vi "dfd_Convert FXP info to MRate Filter.vi"(8 "error in (no error)":errorcluster, 10 "xml string in":string, 11 "multirate filter in":T1={"mMRate_Structure"=enum."CIC", "mMRate_Mode"=0, "mMRate_Factor"=1, "mMRate_FIRParams"={"mMRate_FIR_H"=[], "mMRate_FIR_IsNyquist?"=FALSE, "mMRate_FIR_IsSymmetric?"=FALSE}, "mMRate_CICParams"={"mMRate_CIC_#Stage"=2, "mMRate_CIC_Lag"=1, "mMRate_CIC_Type"=enum."Lowpass"}, "mMRate_Order"=1, "mMRate_Version"="1.0", "mMRate_Comments"="1.0", "mMRate_RationalFactor"={"mMRate_L"=-1, "mMRate_M"=-1}, "mMRate_Fs"=0.0, "mMRate_Quantized?"=FALSE, "mMRate_QFilterGain"=1.0, "mMRate_CoefWl"=16, "mMRate_Scaling"={"mMRate_ScaleByPowerOf2?"=FALSE, "mMRate_ScaleType"=enum."Time Domain 1-Norm"}, "mMRate_InputWl"=0, "mMRate_OutputWl"=0, "mMRate_OutputMode"=enum."Nearest", "mMRate_MultMode"=enum."Truncated", "mMRate_BitPruning"=FALSE, "mMRate_GainWl"=16, "mMRate_OutputFwl"=0, "mMRate_SumIwl"=0, "mMRate_InputIwl "=16, "mMRate_SumWl"=32, "mMRate_CoefIwl"=0} {"mMRate_SumWl" min=1 max=32 step=1; "mMRate_InputIwl" min=1 max=32 step=1; "mMRate_GainWl" min=1 max=32 step=1; "mMRate_OutputWl" min=1 max=32 step=1; "mMRate_InputWl" min=1 max=32 step=1; "mMRate_CoefWl" min=1 max=32 step=1; "mMRate_Mode" items=["Default"=-1, "No Rate Change"=0, "Interpolation"=1, "Decimation"=2, "Interpolated"=3, "Rational"=4]}) -> (0 "error out":errorcluster, 3 "multirate filter out":T1={"mMRate_Structure"=enum."IIR", "mMRate_Mode"=0, "mMRate_Factor"=-1, "mMRate_FIRParams"={"mMRate_FIR_H"=[], "mMRate_FIR_IsNyquist?"=FALSE, "mMRate_FIR_IsSymmetric?"=FALSE}, "mMRate_CICParams"={"mMRate_CIC_#Stage"=0, "mMRate_CIC_Lag"=0, "mMRate_CIC_Type"=enum."Lowpass"}, "mMRate_Order"=0, "mMRate_Version"="2.0", "mMRate_Comments"="", "mMRate_RationalFactor"={"mMRate_L"=-1, "mMRate_M"=-1}, "mMRate_Fs"=1.0, "mMRate_Quantized?"=FALSE, "mMRate_QFilterGain"=1.0, "mMRate_CoefWl"=16, "mMRate_Scaling"={"mMRate_ScaleByPowerOf2?"=FALSE, "mMRate_ScaleType"=enum."No Norm"}, "mMRate_InputWl"=16, "mMRate_OutputWl"=16, "mMRate_OutputMode"=enum."Truncation", "mMRate_MultMode"=enum."Truncated", "mMRate_BitPruning"=FALSE, "mMRate_GainWl"=16, "mMRate_OutputFwl"=0, "mMRate_SumIwl"=0, "mMRate_InputIwl "=16, "mMRate_SumWl"=32, "mMRate_CoefIwl"=0} {"mMRate_SumWl" min=1 max=32 step=1; "mMRate_InputIwl" min=1 max=32 step=1; "mMRate_GainWl" min=1 max=32 step=1; "mMRate_OutputWl" min=1 max=32 step=1; "mMRate_InputWl" min=1 max=32 step=1; "mMRate_CoefWl" min=1 max=32 step=1; "mMRate_Mode" items=["Default"=-1, "No Rate Change"=0, "Interpolation"=1, "Decimation"=2, "Interpolated"=3, "Rational"=4]})   [LabVIEW 2017, in "NI_DigFilter_Process.lvlib"]
uses:
  <vilib>/addons/Digital Filter Design/NI_DigFilter_Process.lvlib
  <vilib>/addons/Digital Filter Design/_Objects.llb/DFD Multirate Filter Obj.ctl
  <vilib>/addons/Digital Filter Design/_Objects.llb/DFD Multirate Mode.ctl
  <vilib>/addons/Digital Filter Design/_Objects.llb/DFD Coef Norm Type.ctl
  <vilib>/addons/Digital Filter Design/_Objects.llb/DFD Round-off Mode.ctl
  <vilib>/addons/Digital Filter Design/_Objects.llb/DFD FXP MRate Multiply Mode.ctl
  <vilib>/addons/Digital Filter Design/_Objects.llb/DFD Quantization Settings.ctl
  <vilib>/addons/Digital Filter Design/_Objects.llb/DFD Quantization Sources.ctl
  <vilib>/addons/Digital Filter Design/FXPLib.llb/DFD I32 to FXP (scalar).vi
  <vilib>/addons/Digital Filter Design/NI_DigFilterLicensed.lvlib
panel:
  in  "Q settings":T6={"source"=0, "wl"=16, "iwl"=1, "overflow mode"=enum."Wrap", "rounding mode"=enum."Truncation", "signed?"=TRUE} {"source" items=["Coefficients a/k"=0, "Coefficients b/v"=7, "Input"=1, "Output"=2, "Multiplicand"=3, "Product"=4, "Sum"=5, "Delay"=6]}
  in  "Q settings":T6={"source"=0, "wl"=16, "iwl"=1, "overflow mode"=enum."Wrap", "rounding mode"=enum."Truncation", "signed?"=TRUE} {"source" items=["Coefficients a/k"=0, "Coefficients b/v"=7, "Input"=1, "Output"=2, "Multiplicand"=3, "Product"=4, "Sum"=5, "Delay"=6]}
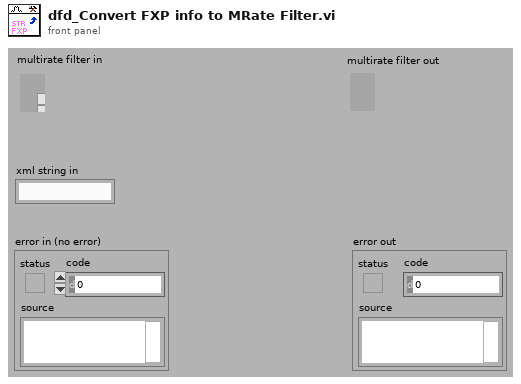
[diagram p1: front panel]
types:
  T1 = typedef "NI_DigFilterLicensed.lvlib/DFD Multirate Filter Obj.ctl" = cluster{"mMRate_Structure":enum16{"CIC", "FIR", "IIR", "Lattice"}, "mMRate_Mode":T2, "mMRate_Factor":i32, "mMRate_FIRParams":cluster{"mMRate_FIR_H":dbl[], "mMRate_FIR_IsNyquist?":bool, "mMRate_FIR_IsSymmetric?":bool}, "mMRate_CICParams":cluster{"mMRate_CIC_#Stage":i32, "mMRate_CIC_Lag":i32, "mMRate_CIC_Type":enum16{"Lowpass", "Highpass"}}, "mMRate_Order":i32, "mMRate_Version":string, "mMRate_Comments":string, "mMRate_RationalFactor":cluster{"mMRate_L":i32, "mMRate_M":i32}, "mMRate_Fs":dbl, "mMRate_Quantized?":bool, "mMRate_QFilterGain":dbl, "mMRate_CoefWl":i16, "mMRate_Scaling":cluster{"mMRate_ScaleByPowerOf2?":bool, "mMRate_ScaleType":T3}, "mMRate_InputWl":i16, "mMRate_OutputWl":i16, "mMRate_OutputMode":T4, "mMRate_MultMode":T5, "mMRate_BitPruning":bool, "mMRate_GainWl":i16, "mMRate_OutputFwl":i16, "mMRate_SumIwl":i16, "mMRate_InputIwl ":i16, "mMRate_SumWl":i16, "mMRate_CoefIwl":i16}
  T2 = typedef "NI_DigFilterLicensed.lvlib/DFD Multirate Mode.ctl" = i16
  T3 = typedef "NI_DigFilterLicensed.lvlib/DFD Coef Norm Type.ctl" = enum16{"No Norm", "Time Domain 1-Norm", "Time Domain 2-Norm", "Time Domain Inf-Norm"}
  T4 = typedef "NI_DigFilterLicensed.lvlib/DFD Round-off Mode.ctl" = enum16{"Nearest", "Truncation"}
  T5 = typedef "NI_DigFilterLicensed.lvlib/DFD FXP MRate Multiply Mode.ctl" = enum16{"Truncated", "Full"}
  T6 = typedef "NI_DigFilterLicensed.lvlib/DFD Quantization Settings.ctl" = cluster{"source":T7, "wl":i16, "iwl":i16, "overflow mode":enum16{"Saturation", "Wrap"}, "rounding mode":enum16{"Nearest", "Truncation"}, "signed?":bool}
  T7 = typedef "NI_DigFilterLicensed.lvlib/DFD Quantization Sources.ctl" = u16
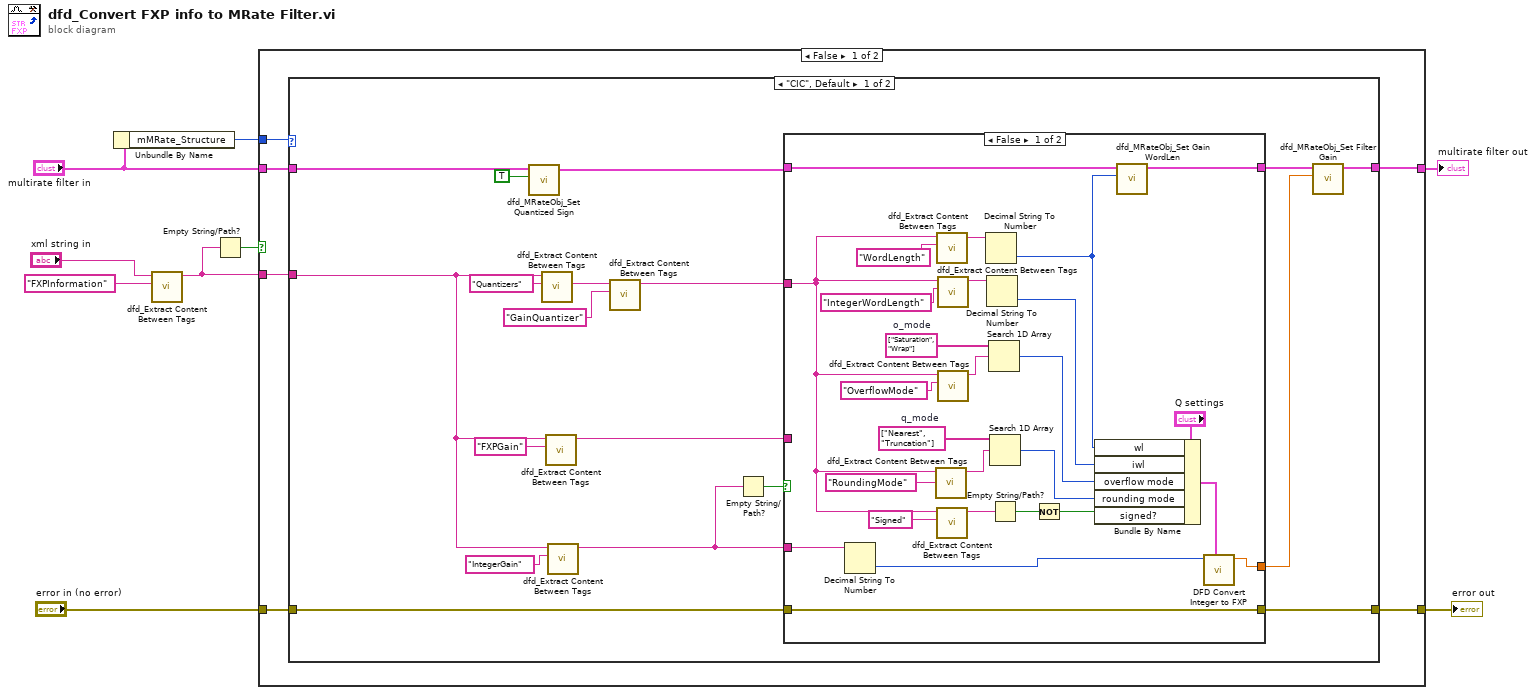
[diagram p0: block diagram]
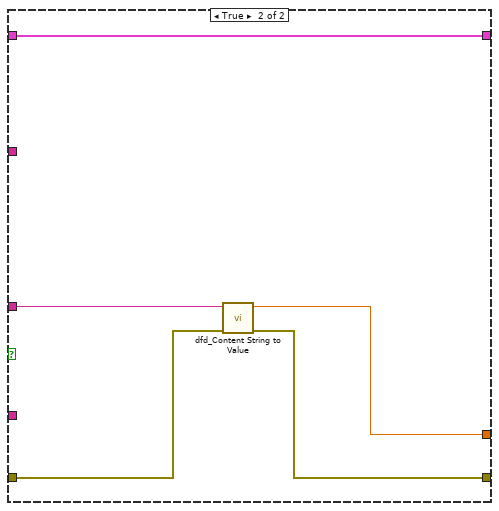
[diagram p2: hidden frame]
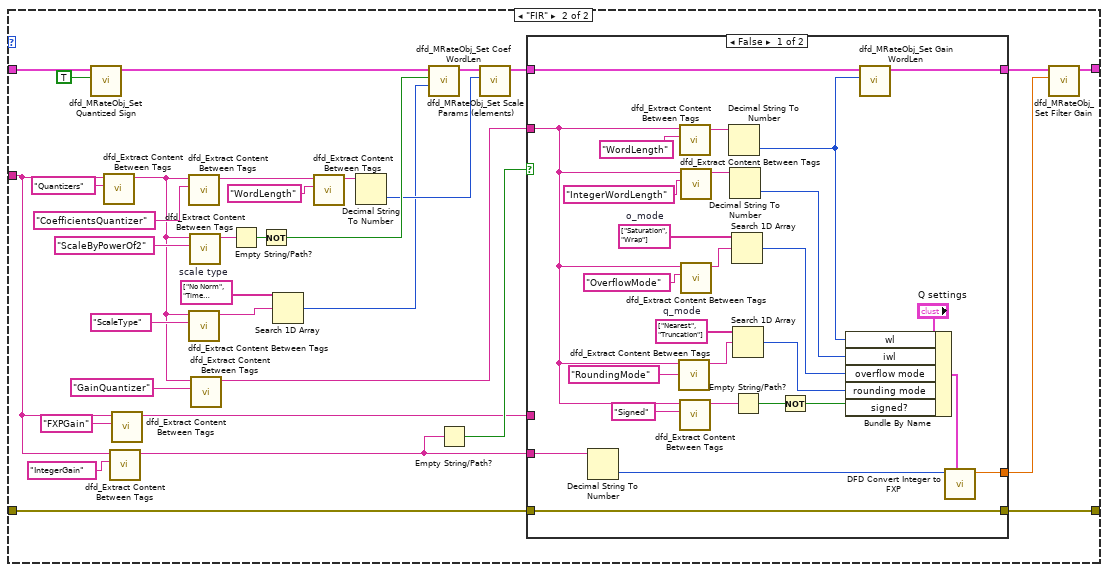
[diagram p3: hidden frame]
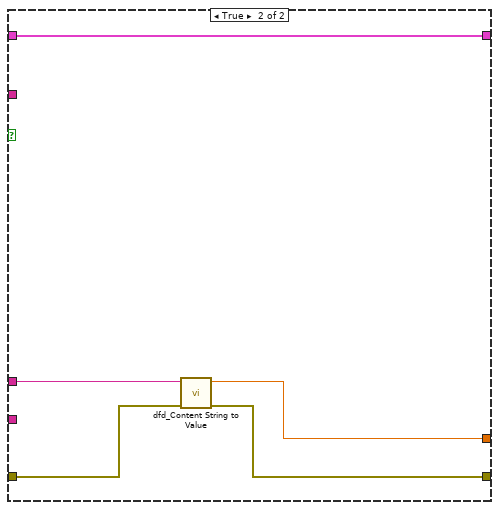
[diagram p4: hidden frame]
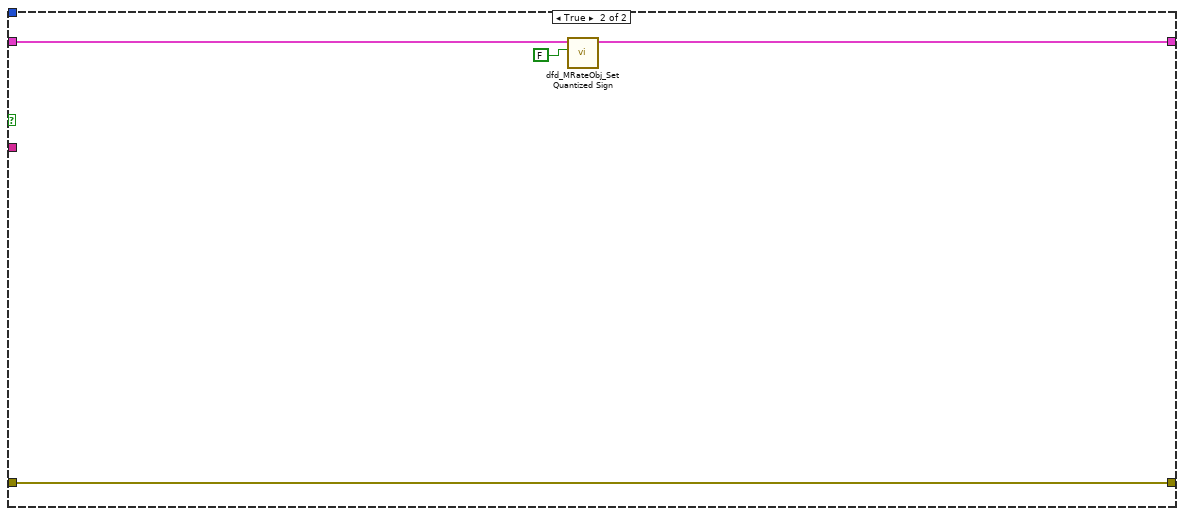
[diagram p5: hidden frame]
diagram:
  n1 = Unbundle By Name("multirate filter in") -> ("mMRate_Structure"=w4:enum16{"CIC", "FIR", "IIR", "Lattice"})
  n2 = call <vilib>:"dfd_Extract Content Between Tags.vi"("element"="FXPInformation", "xml string with tag"="xml string in") -> ("content"=w6:string)  [unwired: 9 out]
  n3 = Empty String/Path?(string/path=w6) -> (empty?=w7:bool)
  n4 = case shown="False" w7 {
    tunnel: "multirate filter in" -> [w13 w133]
    tunnel: w6 -> [w15 _]
    tunnel: w4 -> [w14 _]
    tunnel: [w12 w132] -> w1
    tunnel: "error in (no error)" -> [w11 w131]
    tunnel: [w10 w131] -> w2
    frame False {
      n5 = case shown="\"CIC\", Default" w14 {
        tunnel: w15 -> [w20 w80]
        tunnel: w13 -> [w21 w88]
        tunnel: [w18 w76] -> w12
        tunnel: w11 -> [w17 w75]
        tunnel: [w16 w74] -> w10
        frame "CIC", Default {
          n6 = call <vilib>:"dfd_MRateObj_Set Quantized Sign.vi"("Quantized?"=TRUE, "multirate filter in"=w21) -> ("multirate filter out"=w19:T1)  [unwired: 9 out]
          n7 = call <vilib>:"dfd_Extract Content Between Tags.vi"("element"="Quantizers", "xml string with tag"=w20) -> ("remaining string"=w31:string)  [unwired: 9 out]
          n8 = call <vilib>:"dfd_Extract Content Between Tags.vi"("element"="FXPGain", "xml string with tag"=w20) -> ("content"=w25:string)  [unwired: 9 out]
          n9 = call <vilib>:"dfd_Extract Content Between Tags.vi"("element"="IntegerGain" ("element name"), "xml string with tag"=w20) -> ("content"=w24:string)  [unwired: 9 out]
          n10 = call <vilib>:"dfd_Extract Content Between Tags.vi"("element"="GainQuantizer" ("element name"), "xml string with tag"=w31) -> ("content"=w27:string)  [unwired: 9 out]
          n11 = Empty String/Path?(string/path=w24) -> (empty?=w29:bool)
          n12 = case shown="False" w29 {
            tunnel: w27 -> [w55 _]
            tunnel: w19 -> [w58 w65]
            tunnel: [w57 w65] -> w23
            tunnel: w25 -> [_ w64]
            tunnel: w24 -> [w46 _]
            tunnel: [w38 w63] -> w22
            tunnel: w17 -> [w37 w62]
            tunnel: [w37 w61] -> w16
            frame False {
              w35 = string[] ["Nearest", "Truncation"]  # q_mode
              w36 = string[] ["Saturation", "Wrap"]  # o_mode
              n13 = Decimal String To Number(string=w46) -> (number=w45:i32)  [unwired: 3 out]
              n14 = call <vilib>:"dfd_Extract Content Between Tags.vi"("element"="RoundingMode", "xml string with tag"=w55) -> ("content"=w49:string)  [unwired: 9 out]
              n15 = call <vilib>:"dfd_Extract Content Between Tags.vi"("element"="WordLength", "xml string with tag"=w55) -> ("content"=w59:string)  [unwired: 9 out]
              n16 = call <vilib>:"dfd_Extract Content Between Tags.vi"("element"="Signed", "xml string with tag"=w55) -> ("content"=w48:string)  [unwired: 9 out]
              n17 = call <vilib>:"dfd_Extract Content Between Tags.vi"("element"="IntegerWordLength", "xml string with tag"=w55) -> ("content"=w56:string)  [unwired: 9 out]
              n18 = call <vilib>:"dfd_Extract Content Between Tags.vi"("element"="OverflowMode", "xml string with tag"=w55) -> ("content"=w50:string)  [unwired: 9 out]
              n19 = Decimal String To Number(string=w59) -> (number=w44:i32)  [unwired: 3 out]
              n20 = Decimal String To Number(string=w56) -> (number=w43:i32)  [unwired: 3 out]
              n21 = Search 1D Array(1D array=w36, element=w50) -> (index of element=w42:i32)  [unwired: 1 out]
              n22 = Search 1D Array(1D array=w35, element=w49) -> (index of element=w41:i32)  [unwired: 1 out]
              n23 = Empty String/Path?(string/path=w48) -> (empty?=w40:bool)
              n24 = Not(x=w40) -> (.not. x?=w34:bool)
              n25 = Bundle By Name(cluster="Q settings", "wl"=w44, "iwl"=w43, "overflow mode"=w42, "rounding mode"=w41, "signed?"=w34) -> (w39:T6)
              n26 = call <vilib>:"dfd_MRateObj_Set Gain WordLen.vi"("gain wl"=w44, "multirate filter in"=w58) -> ("multirate filter out"=w57:T1)  [unwired: 9 out]
              n27 = call-poly <vilib>:"DFD Convert Integer to FXP.vi"("quantization settings"=w39, "I32"=w45) -> ("FXP value"=w38:dbl)  [unwired: 1 in, 8 out]
            }
            frame True {
              n28 = call <vilib>:"dfd_Content String to Value.vi"("error in (no error)"=w62, "string"=w64) -> ("error out"=w61:errorcluster, "value"=w63:dbl)  [unwired: 8 out]
            }
          }
          n29 = call <vilib>:"dfd_MRateObj_Set Filter Gain.vi"("gain"=w22, "multirate filter in"=w23) -> ("multirate filter out"=w18:T1)  [unwired: 1 in, 8 out]
        }
        frame "FIR" {
          w66 = string[] ["No Norm", "Time Domain 1-Norm", "Time Domain 2-Norm", "Time Domain Inf-Norm"]  # scale type
          n30 = call <vilib>:"dfd_MRateObj_Set Quantized Sign.vi"("Quantized?"=TRUE, "multirate filter in"=w88) -> ("multirate filter out"=w72:T1)  [unwired: 9 out]
          n31 = call <vilib>:"dfd_Extract Content Between Tags.vi"("element"="Quantizers", "xml string with tag"=w80) -> ("content"=w68:string)  [unwired: 9 out]
          n32 = call <vilib>:"dfd_Extract Content Between Tags.vi"("element"="IntegerGain" ("element name"), "xml string with tag"=w80) -> ("content"=w79:string)  [unwired: 9 out]
          n33 = call <vilib>:"dfd_Extract Content Between Tags.vi"("element"="FXPGain", "xml string with tag"=w80) -> ("content"=w67:string)  [unwired: 9 out]
          n34 = call <vilib>:"dfd_Extract Content Between Tags.vi"("element"="CoefficientsQuantizer" ("element name"), "xml string with tag"=w68) -> ("content"=w86:string)  [unwired: 9 out]
          n35 = call <vilib>:"dfd_Extract Content Between Tags.vi"("element"="ScaleType" ("element name"), "xml string with tag"=w68) -> ("content"=w89:string)  [unwired: 9 out]
          n36 = call <vilib>:"dfd_Extract Content Between Tags.vi"("element"="ScaleByPowerOf2", "xml string with tag"=w68) -> ("content"=w91:string)  [unwired: 9 out]
          n37 = call <vilib>:"dfd_Extract Content Between Tags.vi"("element"="GainQuantizer" ("element name"), "xml string with tag"=w68) -> ("content"=w82:string)  [unwired: 9 out]
          n38 = Empty String/Path?(string/path=w91) -> (empty?=w90:bool)
          n39 = Not(x=w90) -> (.not. x?=w71:bool)
          n40 = Search 1D Array(1D array=w66, element=w89) -> (index of element=w69:i32)  [unwired: 1 out]
          n41 = call <vilib>:"dfd_Extract Content Between Tags.vi"("element"="WordLength", "xml string with tag"=w86) -> ("content"=w84:string)  [unwired: 9 out]
          n42 = Decimal String To Number(string=w84) -> (number=w70:i32)  [unwired: 3 out]
          n43 = call <vilib>:"dfd_MRateObj_Set Scale Params (elements).vi"("scale type"=w69, "scale by Power of 2?"=w71, "multirate filter in"=w72) -> ("multirate filter out"=w83:T1)  [unwired: 8 out]
          n44 = Empty String/Path?(string/path=w79) -> (empty?=w92:bool)
          n45 = call <vilib>:"dfd_MRateObj_Set Coef WordLen.vi"("coef wl"=w70, "multirate filter in"=w83) -> ("multirate filter out"=w73:T1)  [unwired: 9 out]
          n46 = case shown="False" w92 {
            tunnel: w82 -> [w120 _]
            tunnel: w73 -> [w123 w130]
            tunnel: [w122 w130] -> w78
            tunnel: w67 -> [_ w129]
            tunnel: w79 -> [w111 _]
            tunnel: [w103 w128] -> w77
            tunnel: w75 -> [w102 w127]
            tunnel: [w102 w126] -> w74
            frame False {
              w100 = string[] ["Nearest", "Truncation"]  # q_mode
              w101 = string[] ["Saturation", "Wrap"]  # o_mode
              n47 = Decimal String To Number(string=w111) -> (number=w110:i32)  [unwired: 3 out]
              n48 = call <vilib>:"dfd_Extract Content Between Tags.vi"("element"="RoundingMode", "xml string with tag"=w120) -> ("content"=w114:string)  [unwired: 9 out]
              n49 = call <vilib>:"dfd_Extract Content Between Tags.vi"("element"="WordLength", "xml string with tag"=w120) -> ("content"=w124:string)  [unwired: 9 out]
              n50 = call <vilib>:"dfd_Extract Content Between Tags.vi"("element"="Signed", "xml string with tag"=w120) -> ("content"=w113:string)  [unwired: 9 out]
              n51 = call <vilib>:"dfd_Extract Content Between Tags.vi"("element"="IntegerWordLength", "xml string with tag"=w120) -> ("content"=w121:string)  [unwired: 9 out]
              n52 = call <vilib>:"dfd_Extract Content Between Tags.vi"("element"="OverflowMode", "xml string with tag"=w120) -> ("content"=w115:string)  [unwired: 9 out]
              n53 = Decimal String To Number(string=w124) -> (number=w109:i32)  [unwired: 3 out]
              n54 = Decimal String To Number(string=w121) -> (number=w108:i32)  [unwired: 3 out]
              n55 = Search 1D Array(1D array=w101, element=w115) -> (index of element=w107:i32)  [unwired: 1 out]
              n56 = Search 1D Array(1D array=w100, element=w114) -> (index of element=w106:i32)  [unwired: 1 out]
              n57 = Empty String/Path?(string/path=w113) -> (empty?=w105:bool)
              n58 = Not(x=w105) -> (.not. x?=w99:bool)
              n59 = Bundle By Name(cluster="Q settings", "wl"=w109, "iwl"=w108, "overflow mode"=w107, "rounding mode"=w106, "signed?"=w99) -> (w104:T6)
              n60 = call <vilib>:"dfd_MRateObj_Set Gain WordLen.vi"("gain wl"=w109, "multirate filter in"=w123) -> ("multirate filter out"=w122:T1)  [unwired: 9 out]
              n61 = call-poly <vilib>:"DFD Convert Integer to FXP.vi"("quantization settings"=w104, "I32"=w110) -> ("FXP value"=w103:dbl)  [unwired: 1 in, 8 out]
            }
            frame True {
              n62 = call <vilib>:"dfd_Content String to Value.vi"("error in (no error)"=w127, "string"=w129) -> ("error out"=w126:errorcluster, "value"=w128:dbl)  [unwired: 8 out]
            }
          }
          n63 = call <vilib>:"dfd_MRateObj_Set Filter Gain.vi"("gain"=w77, "multirate filter in"=w78) -> ("multirate filter out"=w76:T1)  [unwired: 1 in, 8 out]
        }
      }
    }
    frame True {
      n64 = call <vilib>:"dfd_MRateObj_Set Quantized Sign.vi"("Quantized?"=FALSE, "multirate filter in"=w133) -> ("multirate filter out"=w132:T1)  [unwired: 9 out]
    }
  }
  "error out" <- w2
  "multirate filter out" <- w1
